vi "ExtraTreesClassifier.vi"(8 "error in":errorcluster) -> (0 "error out":errorcluster, 3 "out":refnum<class "ExtraTreesClassifier.lvclass">)   [LabVIEW 2020]
doc: "An extra-trees classifier.\n\n This class implements a meta estimator that fits a number of\n randomized decision trees (a.k.a. extra-trees) on various sub-samples\n of the dataset and uses averaging to improve the predictive accuracy\n and control over-fitting.\n\n Read more in the :ref:`User Guide <forest>`.\n\n Parameters\n ----------\n n_estimators : int, default=100\n The number of trees in the forest.\n\n .. versionchanged:: 0.22\n The default value of ``n_estimators`` changed from 10 to 100\n in 0.22.\n\n criterion : {\"gini\", \"entropy\"}, default=\"gini\"\n The function to measure the quality of a split. Supported criteria are\n \"gini\" for the Gini impurity and \"entropy\" for the information gain.\n\n max_depth : int, default=None\n The maximum depth of the tree. If None, then nodes are expanded until\n all leaves are pure or until all leaves contain less than\n min_samples_split samples.\n\n min_samples_split : int or float, default=2\n The minimum number of samples required to split an internal node:\n\n - If int, then consider `min_samples_split` as the minimum number.\n - If float, then `min_samples_split` is a fraction and\n `ceil(min_samples_split * n_samples)` are the minimum\n number of samples for each split.\n\n .. versionchanged:: 0.18\n Added float values for fractions.\n\n min_samples_leaf : int or float, default=1\n The minimum number of samples required to be at a leaf node.\n A split point at any depth will only be considered if it leaves at\n least ``min_samples_leaf`` training samples in each of the left and\n right branches. This may have the effect of smoothing the model,\n especially in regression.\n\n - If int, then consider `min_samples_leaf` as the minimum number.\n - If float, then `min_samples_leaf` is a fraction and\n `ceil(min_samples_leaf * n_samples)` are the minimum\n number of samples for each node.\n\n .. versionchanged:: 0.18\n Added float values for fractions.\n\n min_weight_fraction_leaf : float, default=0.0\n The minimum weighted fraction of the sum total of weights (of all\n the input samples) required to be at a leaf node. Samples have\n equal weight when sample_weight is not provided.\n\n max_features : {\"auto\", \"sqrt\", \"log2\"}, int or float, default=\"auto\"\n The number of features to consider when looking for the best split:\n\n - If int, then consider `max_features` features at each split.\n - If float, then `max_features` is a fraction and\n `round(max_features * n_features)` features are considered at each\n split.\n - If \"auto\", then `max_features=sqrt(n_features)`.\n - If \"sqrt\", then `max_features=sqrt(n_features)`.\n - If \"log2\", then `max_features=log2(n_features)`.\n - If None, then `max_features=n_features`.\n\n Note: the search for a split does not stop until at least one\n valid partition of the node samples is found, even if it requires to\n effectively inspect more than ``max_features`` features.\n\n max_leaf_nodes : int, default=None\n Grow trees with ``max_leaf_nodes`` in best-first fashion.\n Best nodes are defined as relative reduction in impurity.\n If None then unlimited number of leaf nodes.\n\n min_impurity_decrease : float, default=0.0\n A node will be split if this split induces a decrease of the impurity\n greater than or equal to this value.\n\n The weighted impurity decrease equation is the following::\n\n N_t / N * (impurity - N_t_R / N_t * right_impurity\n - N_t_L / N_t * left_impurity)\n\n where ``N`` is the total number of samples, ``N_t`` is the number of\n samples at the current node, ``N_t_L`` is the number of samples in the\n left child, and ``N_t_R`` is the number of samples in the right child.\n\n ``N``, ``N_t``, ``N_t_R`` and ``N_t_L`` all refer to the weighted sum,\n if ``sample_weight`` is passed.\n\n .. versionadded:: 0.19\n\n min_impurity_split : float, default=None\n Threshold for early stopping in tree growth. A node will split\n if its impurity is above the threshold, otherwise it is a leaf.\n\n .. deprecated:: 0.19\n ``min_impurity_split`` has been deprecated in favor of\n ``min_impurity_decrease`` in 0.19. The default value of\n ``min_impurity_split`` has changed from 1e-7 to 0 in 0.23 and it\n will be removed in 1.0 (renaming of 0.25).\n Use ``min_impurity_decrease`` instead.\n\n bootstrap : bool, default=False\n Whether bootstrap samples are used when building trees. If False, the\n whole dataset is used to build each tree.\n\n oob_score : bool, default=False\n Whether to use out-of-bag samples to estimate the generalization score.\n Only available if bootstrap=True.\n\n n_jobs : int, default=None\n The number of jobs to run in parallel. :meth:`fit`, :meth:`predict`,\n :meth:`decision_path` and :meth:`apply` are all parallelized over the\n trees. ``None`` means 1 unless in a :obj:`joblib.parallel_backend`\n context. ``-1`` means using all processors. See :term:`Glossary\n <n_jobs>` for more details.\n\n random_state : int, RandomState instance or None, default=None\n Controls 3 sources of randomness:\n\n - the bootstrapping of the samples used when building trees\n (if ``bootstrap=True``)\n - the sampling of the features to consider when looking for the best\n split at each node (if ``max_features < n_features``)\n - the draw of the splits for each of the `max_features`\n\n See :term:`Glossary <random_state>` for details.\n\n verbose : int, default=0\n Controls the verbosity when fitting and predicting.\n\n warm_start : bool, default=False\n When set to ``True``, reuse the solution of the previous call to fit\n and add more estimators to the ensemble, otherwise, just fit a whole\n new forest. See :term:`the Glossary <warm_start>`.\n\n class_weight : {\"balanced\", \"balanced_subsample\"}, dict or list of dicts, default=None\n Weights associated with classes in the form ``{class_label: weight}``.\n If not given, all classes are supposed to have weight one. For\n multi-output problems, a list of dicts can be provided in the same\n order as the columns of y.\n\n Note that for multioutput (including multilabel) weights should be\n defined for each class of every column in its own dict. For example,\n for four-class multilabel classification weights should be\n [{0: 1, 1: 1}, {0: 1, 1: 5}, {0: 1, 1: 1}, {0: 1, 1: 1}] instead of\n [{1:1}, {2:5}, {3:1}, {4:1}].\n\n The \"balanced\" mode uses the values of y to automatically adjust\n weights inversely proportional to class frequencies in the input data\n as ``n_samples / (n_classes * np.bincount(y))``\n\n The \"balanced_subsample\" mode is the same as \"balanced\" except that\n weights are computed based on the bootstrap sample for every tree\n grown.\n\n For multi-output, the weights of each column of y will be multiplied.\n\n Note that these weights will be multiplied with sample_weight (passed\n through the fit method) if sample_weight is specified.\n\n ccp_alpha : non-negative float, default=0.0\n Complexity parameter used for Minimal Cost-Complexity Pruning. The\n subtree with the largest cost complexity that is smaller than\n ``ccp_alpha`` will be chosen. By default, no pruning is performed. See\n :ref:`minimal_cost_complexity_pruning` for details.\n\n .. versionadded:: 0.22\n\n max_samples : int or float, default=None\n If bootstrap is True, the number of samples to draw from X\n to train each base estimator.\n\n - If None (default), then draw `X.shape[0]` samples.\n - If int, then draw `max_samples` samples.\n - If float, then draw `max_samples * X.shape[0]` samples. Thus,\n `max_samples` should be in the interval `(0, 1)`.\n\n .. versionadded:: 0.22\n\n Attributes\n ----------\n base_estimator_ : ExtraTreesClassifier\n The child estimator template used to create the collection of fitted\n sub-estimators.\n\n estimators_ : list of DecisionTreeClassifier\n The collection of fitted sub-estimators.\n\n classes_ : ndarray of shape (n_classes,) or a list of such arrays\n The classes labels (single output problem), or a list of arrays of\n class labels (multi-output problem).\n\n n_classes_ : int or list\n The number of classes (single output problem), or a list containing the\n number of classes for each output (multi-output problem).\n\n feature_importances_ : ndarray of shape (n_features,)\n The impurity-based feature importances.\n The higher, the more important the feature.\n The importance of a feature is computed as the (normalized)\n total reduction of the criterion brought by that feature. It is also\n known as the Gini importance.\n\n Warning: impurity-based feature importances can be misleading for\n high cardinality features (many unique values). See\n :func:`sklearn.inspection.permutation_importance` as an alternative.\n\n n_features_ : int\n The number of features when ``fit`` is performed.\n\n n_outputs_ : int\n The number of outputs when ``fit`` is performed.\n\n oob_score_ : float\n Score of the training dataset obtained using an out-of-bag estimate.\n This attribute exists only when ``oob_score`` is True.\n\n oob_decision_function_ : ndarray of shape (n_samples, n_classes)\n Decision function computed with out-of-bag estimate on the training\n set. If n_estimators is small it might be possible that a data point\n was never left out during the bootstrap. In this case,\n `oob_decision_function_` might contain NaN. This attribute exists\n only when ``oob_score`` is True.\n\n See Also\n --------\n sklearn.tree.ExtraTreeClassifier : Base classifier for this ensemble.\n RandomForestClassifier : Ensemble Classifier based on trees with optimal\n splits.\n\n Notes\n -----\n The default values for the parameters controlling the size of the trees\n (e.g. ``max_depth``, ``min_samples_leaf``, etc.) lead to fully grown and\n unpruned trees which can potentially be very large on some data sets. To\n reduce memory consumption, the complexity and size of the trees should be\n controlled by setting those parameter values.\n\n References\n ----------\n .. [1] P. Geurts, D. Ernst., and L. Wehenkel, \"Extremely randomized\n trees\", Machine Learning, 63(1), 3-42, 2006.\n\n \nAvailable methods:\nPredict Log Proba\nPredict Proba\nFit\nPredict\nScore\nGet Attributes\nGet Params\nSet Params"
uses:
  ExtraTreesClassifier.lvclass
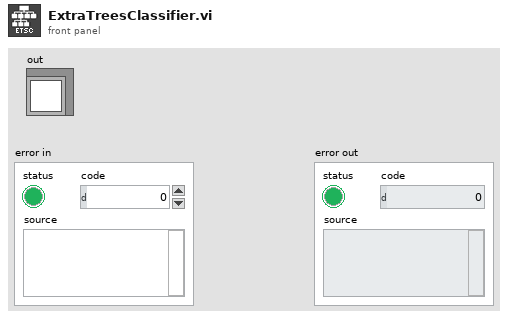
[diagram p1: front panel]
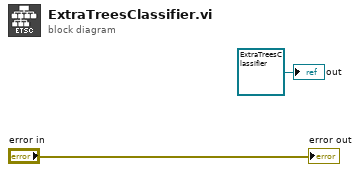
[diagram p0: block diagram]
diagram:
  "out" <- refnum<class "ExtraTreesClassifier.lvclass"> refnum ("model")
  "error out" <- "error in"
